vi "createDocument.vi"(8 "error in (no error)":errorcluster, 11 "MS-Word in":refnum<class "MS-Word.lvclass">) -> (0 "error out":errorcluster, 3 "MS-Word out":refnum<class "MS-Word.lvclass">)   [LabVIEW 2017, in "LabVIEW NPOI.lvlib" / "MS-Word.lvclass"]
doc: "Protected dynamic dispatch method to create a new <b>Document</b> at the <b>File Path</b> location. Use save to persist your changes."
uses:
  MS-Word.lvclass
  C:/Users/Neo/Desktop/Dev_Tools_BR/LabVIEW_NPOI/src/LabVIEW NPOI/Document/Document.lvclass
  Document/Document.lvclass/Document.ctl
  Document/Get FilePath.vi
  xwpfDocument/xwpfDocument.lvclass
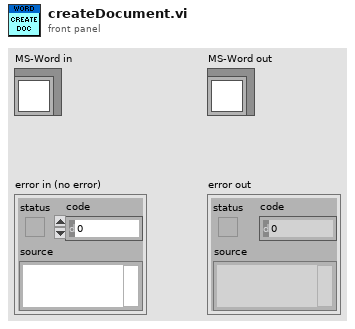
[diagram p1: front panel]
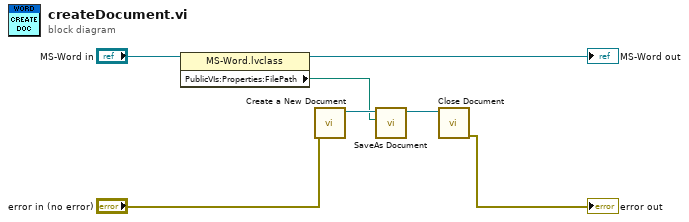
[diagram p0: block diagram]
diagram:
  n1 = property class="MS-Word.lvclass"(reference="MS-Word in") -> (reference out=→"MS-Word out":refnum<class "MS-Word.lvclass">, "PublicVIs:Properties:FilePath"=w1:path)  [unwired: 1 in, 1 out]
  n2 = call "Create a New Document.vi"("error in (no error)"="error in (no error)") -> ("xwpfDocument out"=w4:refnum<class "xwpfDocument.lvclass">)  [unwired: 9 in, 1 out]
  n3 = call "SaveAs Document.vi"("Document Path"=w1, "xwpfDocument in"=w4) -> ("xwpfDocument out"=w2:refnum<class "xwpfDocument.lvclass">)  [unwired: 8 in, 1 out]
  n4 = call "Close Document.vi"("xwpfDocument in"=w2) -> ("error out"=→"error out":errorcluster)  [unwired: 9 in, 1 out]
